vi "_setRef.vi"(7 "parentURL":string, 8 "error in (no error)":errorcluster, 9 "Name":string, 10 "Refnum":variant, 11 "TagDB in":T1) -> (0 "error out":errorcluster, 2 "URL":string, 3 "TagDB out":T1)   [LabVIEW 2014, in "RefManager(dev).lvlib"]
uses:
  RefManager(dev).lvlib
  <userlib>/_NEVSTOP/TagDB/Core/tagDB_Def.ctl
  <userlib>/_NEVSTOP/TagDB/Core/TagDB.lvlib
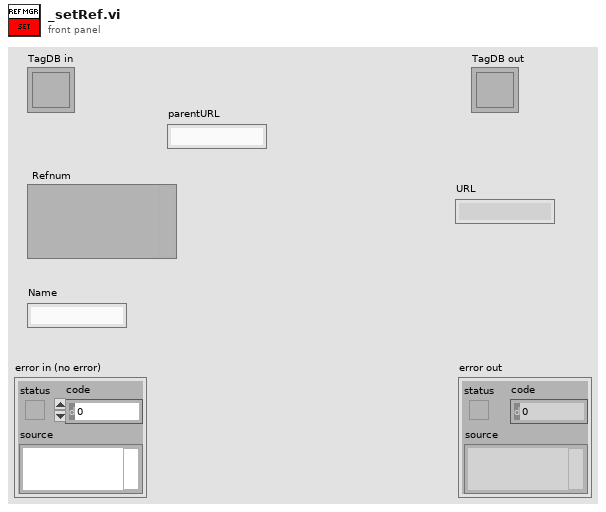
[diagram p1: front panel]
types:
  T1 = typedef "TagDB.lvlib/tagDB_Def.ctl" = refnum<k1>
  T2 = enum8{"<Null>", "I8", "I16", "I32", "I64", "U8", "U16", "U32", "U64", "SGL", "DBL", "EXT", "CSG", "CDB", "CXT", "0x0F", "0x10", "0x11", "0x12", "0x13", "0x14", "Enum U8", "Enum U16", "Enum U32", "Enum U64", "SGL PQ", "DBL PQ", "EXT PQ", "CSG PQ", "CDB PQ", "CXT PQ", "0x1F", "0x20", "Boolean", "0x22", "0x23", "0x24", "0x25", "0x26", "0x27", "0x28", "0x29", "0x2A", "0x2B", "0x2C", "0x2D", "0x2E", "0x2F", "String", "0x31", "Path", "Pict", "0x34", "0x35", "0x36", "DAQ", "0x38", "0x39", "0x3A", "0x3B", "0x3C", "0x3D", "0x3E", "0x3F", "Array", "0x41", "0x42", "0x43", "0x44", "0x45", "0x46", "0x47", "0x48", "0x49", "0x4A", "0x4B", "0x4C", "0x4D", "0x4E", "0x4F", "Cluster", "0x51", "0x52", "Variant", "Waveform", "0x55", "0x56", "0x57", "0x58", "0x59", "0x5A", "0x5B", "0x5C", "0x5D", "0x5E", "0x5F", "0x60", "0x61", "0x62", "0x63", "0x64", "0x65", "0x66", "0x67", "0x68", "0x69", "0x6A", "0x6B", "0x6C", "0x6D", "0x6E", "0x6F", "Refnum"}
  T3 = enum8{"Generic", "Datalog File Refnum", "Byte Stream File Refnum", "Device Refnum", "Occurence Refnum", "TCP Connection Refnum", "VISA Refnum (Obsolete)", "Automation Renum", "VI Server Refnum", "Menu Refnum", "IVI Refnum (Obsolete)", "IMAQ Session", "0x0C", "Datasocket Refnum", "VISA Resource", "IVI Logical Name", "UDP Connection Refnum", "Notifier Refnum", "Queue Refnum", "IrDA Refnum", "Hardware Plugin Refnum", "Hardware Plugin Tag Refnum", "DAQmx Refnum", "Event Registration Refnum", ".NET Refnum", "User Event Refnum", "0x1A", "Event Callback", "0x1C", "0x1D", "Only Used Internal to LabVIEW", "Bluetooth", "Data Value References", "RT FIFO", "TDM Streaming"}
  T4 = enum16{"Not a VI Server Refnum", "Control", "VI", "Application", "Splitter", "Pane"}
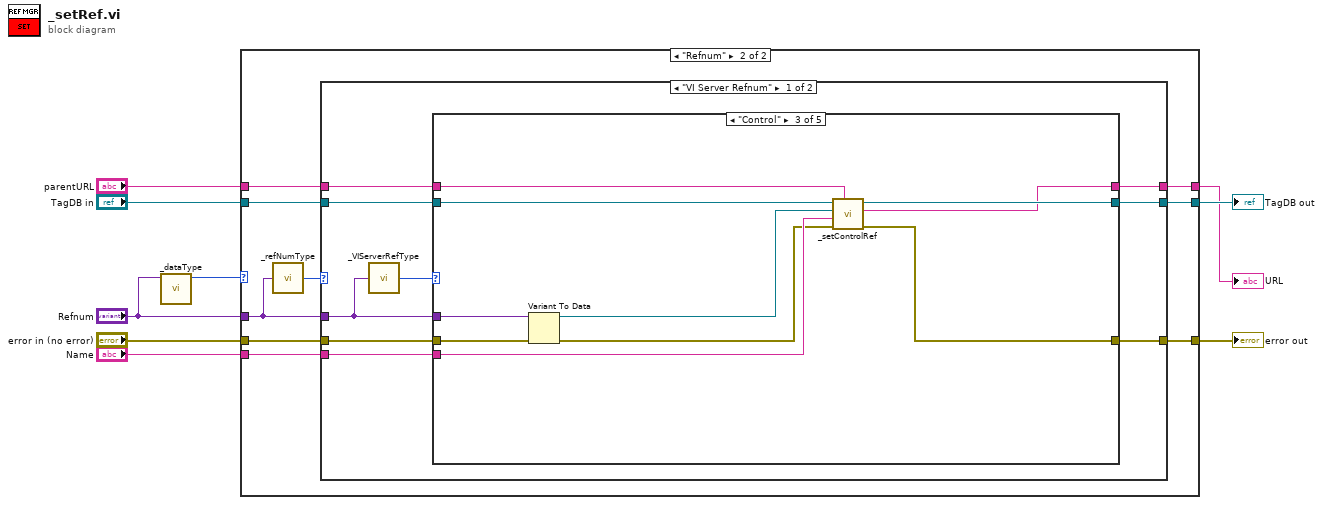
[diagram p0: block diagram]
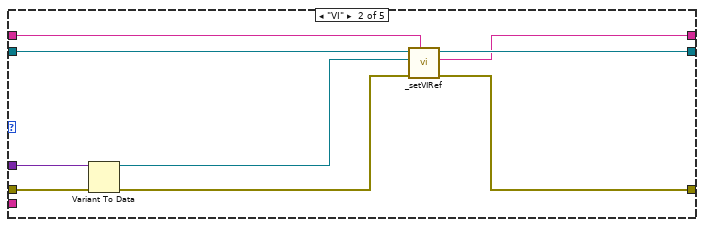
[diagram p4: hidden frame]
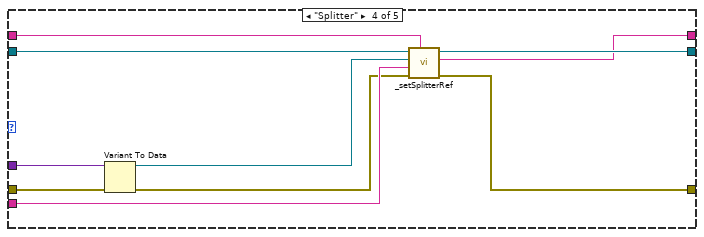
[diagram p5: hidden frame]
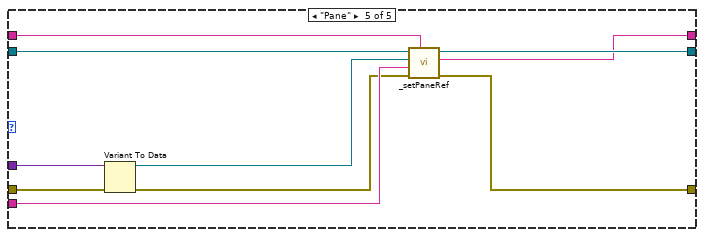
[diagram p6: hidden frame]
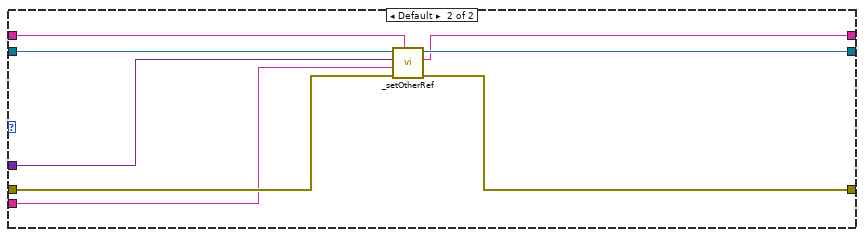
[diagram p7: hidden frame]
diagram:
  n1 = call <userlib>:"_dataType.vi"("Type"="Refnum") -> ("type"=w9:T2)  [unwired: 10 in]
  n2 = case shown="\"Refnum\"" w9 {
    tunnel: [w12 w20] -> w8
    tunnel: "TagDB in" -> [w12 w19]
    tunnel: [w11 w18] -> w6
    tunnel: "error in (no error)" -> [w11 w17]
    tunnel: "Refnum" -> [_ w16]
    tunnel: "parentURL" -> [w10 w15]
    tunnel: "Name" -> [_ w14]
    tunnel: [w10 w13] -> w1
    frame Default {
    }
    frame "Refnum" {
      n3 = call <userlib>:"_refNumType.vi"("Data"=w16) -> ("Refnum Subtype Enum"=w21:T3)  [unwired: 4 in]
      n4 = case shown="\"VI Server Refnum\"" w21 {
        tunnel: [w30 w79] -> w20
        tunnel: w19 -> [w29 w80]
        tunnel: [w27 w76] -> w18
        tunnel: w17 -> [w26 w77]
        tunnel: w16 -> [w23 w74]
        tunnel: w15 -> [w25 w78]
        tunnel: w14 -> [w24 w75]
        tunnel: [w22 w73] -> w13
        frame "VI Server Refnum" {
          n5 = call <userlib>:"_VIServerRefType.vi"("Data"=w23) -> ("Enum"=w28:T4)  [unwired: 4 in]
          n6 = case shown="\"Control\"" w28 {
            tunnel: [w33 w40 w50 w60 w70] -> w30
            tunnel: w29 -> [w33 w42 w52 w62 w72]
            tunnel: [w32 w39 w49 w59 w69] -> w27
            tunnel: w26 -> [w32 w36 w45 w55 w65]
            tunnel: w25 -> [w31 w41 w51 w61 w71]
            tunnel: w24 -> [_ _ w48 w58 w68]
            tunnel: w23 -> [_ w38 w47 w57 w67]
            tunnel: [w31 w34 w43 w53 w63] -> w22
            frame "Not a VI Server Refnum", Default {
            }
            frame "VI" {
              n7 = Variant To Data(error in=w36, Variant=w38) -> (data=w37:refnum<vi>, error out=w35:errorcluster)  [unwired: 1 in]
              n8 = call "_setVIRef.vi"("parentURL"=w41, "error in (no error)"=w35, "Refnum"=w37, "TagDB in"=w42) -> ("error out"=w39:errorcluster, "URL"=w34:string, "TagDB out"=w40:T1)  [unwired: 5 in]
            }
            frame "Control" {
              n9 = Variant To Data(error in=w45, Variant=w47) -> (data=w46:refnum<vi>, error out=w44:errorcluster)  [unwired: 1 in]
              n10 = call "_setControlRef.vi"("parentURL"=w51, "error in (no error)"=w44, "Name"=w48, "Refnum"=w46, "TagDB in"=w52) -> ("error out"=w49:errorcluster, "Ref-Key"=w43:string, "TagDB out"=w50:T1)  [unwired: 4 in]
            }
            frame "Splitter" {
              n11 = Variant To Data(error in=w55, Variant=w57) -> (data=w56:refnum<vi>, error out=w54:errorcluster)  [unwired: 1 in]
              n12 = call "_setSplitterRef.vi"("parentURL"=w61, "error in (no error)"=w54, "Name"=w58, "Refnum"=w56, "TagDB in"=w62) -> ("error out"=w59:errorcluster, "URL"=w53:string, "TagDB out"=w60:T1)  [unwired: 4 in]
            }
            frame "Pane" {
              n13 = Variant To Data(error in=w65, Variant=w67) -> (data=w66:refnum<vi>, error out=w64:errorcluster)  [unwired: 1 in]
              n14 = call "_setPaneRef.vi"("parentURL"=w71, "error in (no error)"=w64, "Name"=w68, "Refnum"=w66, "TagDB in"=w72) -> ("error out"=w69:errorcluster, "URL"=w63:string, "TagDB out"=w70:T1)  [unwired: 4 in]
            }
          }
        }
        frame Default {
          n15 = call "_setOtherRef.vi"("parentURL"=w78, "error in (no error)"=w77, "Name"=w75, "Refnum"=w74, "TagDB in"=w80) -> ("error out"=w76:errorcluster, "Ref-Key"=w73:string, "TagDB out"=w79:T1)  [unwired: 4 in]
        }
      }
    }
  }
  "error out" <- w6
  "TagDB out" <- w8
  "URL" <- w1
